vi "Display Console View.vi"(8 "error in (no error)":errorcluster, 11 "View Model":T2) -> (0 "error out":errorcluster)   [LabVIEW 2017]
doc: "Display console for debugging elevator operation"
uses:
  View Model/Controls/View Model.ctl
  Error Handler/Controls/Error Model.ctl
  Error Handler/Controls/Error Type.ctl
  View Model/Controls/Shared Model.ctl
  Elevator Controller/Controls/Elevator Model.ctl
  Elevator Controller/Controls/Controller Overhead.ctl
panel:
  out "Elevator Location":T1(ring)
  out "Down":bool
  out "Emergency":bool
  out "Door Open":bool
  out "Up":bool
  out "Timing":dbl
  # "Elevator Direction"
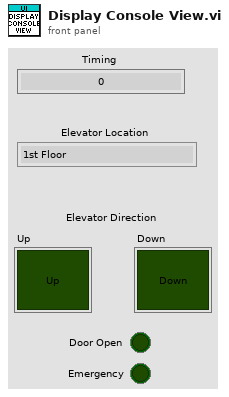
[diagram p1: front panel]
types:
  T1 = enum16{"1st Floor", "2nd Floor", "3rd Floor", "4th Floor"}
  T2 = typedef "View Model.ctl" = cluster{"Error Model":T3, "Shared Model":T4, "Elevator Model":T5}
  T3 = typedef "Error Model.ctl" = cluster{"Error Event":refnum<user-event>}
  T4 = typedef "Shared Model.ctl" = cluster{"Stop DVR":refnum<data-value>, "Stop Event":refnum<user-event>}
  T5 = typedef "Elevator Model.ctl" = cluster{"Controller Overhead":refnum<data-value>, "Motion Change":refnum<user-event>, "Direction Change":refnum<user-event>, "Door Position Change":refnum<user-event>, "Emergency Change":refnum<user-event>, "Floor Change":refnum<user-event>}
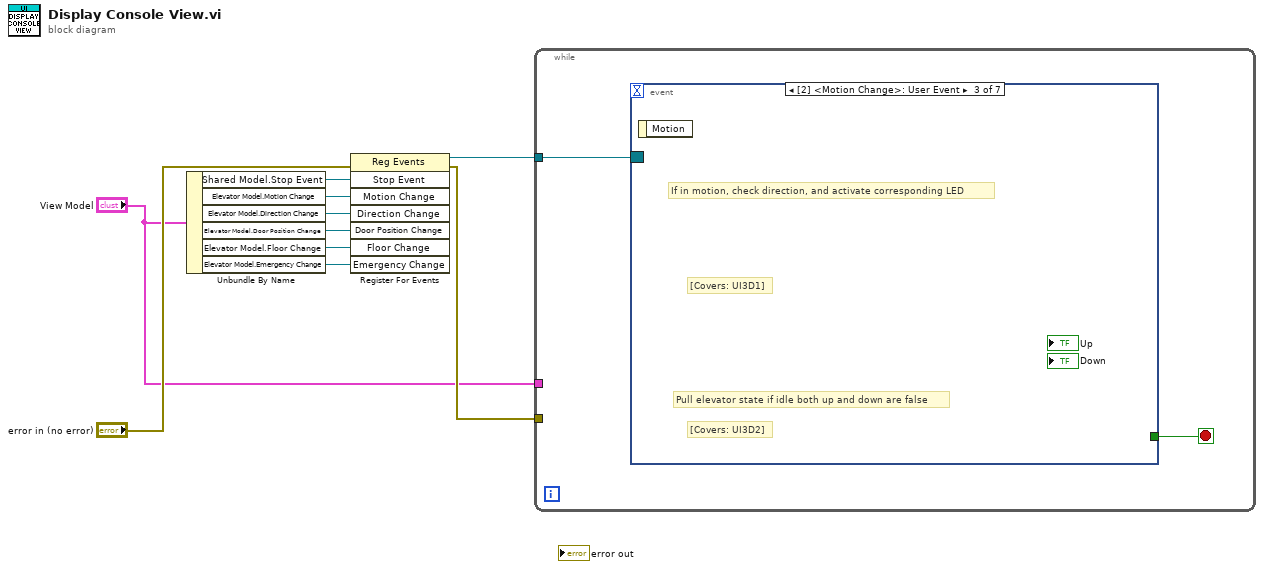
[diagram p0: block diagram]
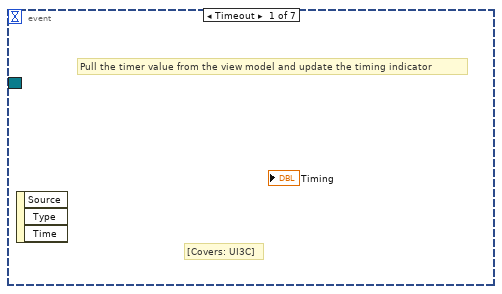
[diagram p2: hidden frame]
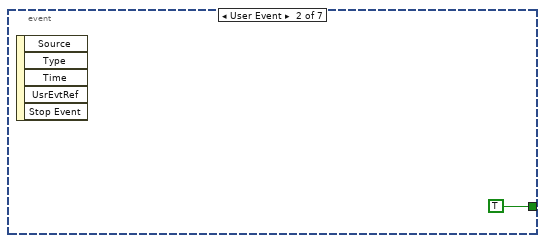
[diagram p3: hidden frame]
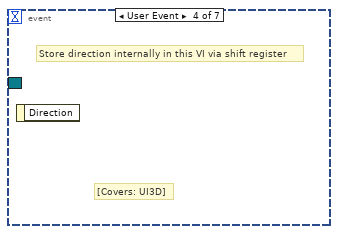
[diagram p4: hidden frame]
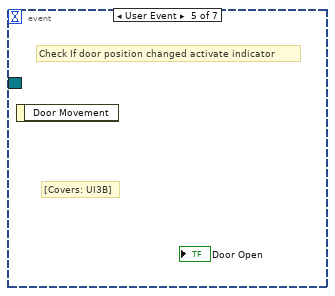
[diagram p5: hidden frame]
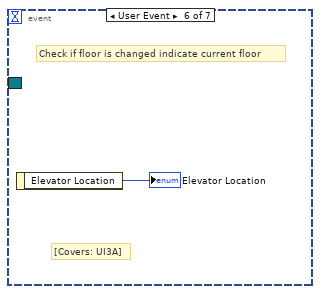
[diagram p6: hidden frame]
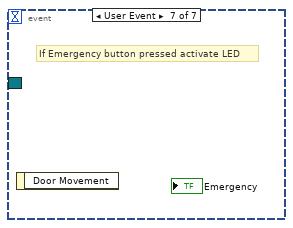
[diagram p7: hidden frame]
diagram:
  n1 = Unbundle By Name("View Model") -> ("Shared Model.Stop Event"=w10:refnum<user-event>, "Elevator Model.Motion Change"=w9:refnum<user-event>, "Elevator Model.Direction Change"=w8:refnum<user-event>, "Elevator Model.Door Position Change"=w7:refnum<user-event>, "Elevator Model.Floor Change"=w2:refnum<user-event>, "Elevator Model.Emergency Change"=w1:refnum<user-event>)
  n2 = register-events(error in="error in (no error)", w10, w9, w8, w7, w2, w1) -> (reference out=w6:refnum<event-registration>, error out=w4:errorcluster)  [unwired: 1 in]
  n3 = while {
    tunnel: w6 -> [w12]
    tunnel: w4 -> [_]
    tunnel: "View Model" -> [_]
    stop <- w11 stop-if-true
    n4 = event shown="[2] <Motion Change>: User Event" {
      selector: w12 -> [_ _ _ _ _ _ _]
      dyn-events: _ -> [_ _ _ _ _ _ _]
      timeout: _ -> [_ _ _ _ _ _ _]
      tunnel: [_ TRUE _ _ _ _ _] -> w11
      event Timeout {
        # "[Covers: UI3C]"
        # "Pull the timer value from the view model and update the timing indicator"
        n5 = event-data() -> ()  [unwired: 1 in, 3 out]
      }
      event User Event {
        n6 = event-data() -> ()  [unwired: 1 in, 5 out]
      }
      event User Event {
        # "[Covers: UI3D2]"
        # "Pull elevator state if idle both up and down are false"
        # "[Covers: UI3D1]"
        # "If in motion, check direction, and activate corresponding LED"
        n7 = event-data() -> ()  [unwired: 1 in, 1 out]
      }
      event User Event {
        # "[Covers: UI3D]"
        # "Store direction internally in this VI via shift register"
        n8 = event-data() -> ()  [unwired: 1 in, 1 out]
      }
      event User Event {
        # "[Covers: UI3B]"
        # "Check If door position changed activate indicator"
        n9 = event-data() -> ()  [unwired: 1 in, 1 out]
      }
      event User Event {
        # "[Covers: UI3A]"
        # "Check if floor is changed indicate current floor"
        n10 = event-data() -> ("Elevator Location"=→"Elevator Location":T1)  [unwired: 1 in]
      }
      event User Event {
        # "If Emergency button pressed activate LED"
        n11 = event-data() -> ()  [unwired: 1 in, 1 out]
      }
    }
  }
